vi "laneleftright411_temp.vi"() -> ()   [LabVIEW 2015]
uses:
  <vilib>/Analysis/6fits.llb/Curve Fitting Criteria.ctl
  <vilib>/Analysis/1siggen.llb/Ramp Pattern by Samples.vi
  <vilib>/Analysis/1siggen.llb/Ramp Pattern by Delta.vi
  G_ALL.vi
  <vilib>/Analysis/polynomials.llb/nth Derivative of Polynomial (DBL).vi
  <vilib>/Analysis/polynomials.llb/1D Polynomial Evaluation (DBL).vi
  G_LCM.vi
  <vilib>/Analysis/NI_AALBase.lvlib
  <vilib>/Analysis/NI_AALPro.lvlib
panel:
  out "y_ramp":dbl[](array[numeric])
  out "y_car":dbl[](array[numeric])
  out "x_car":dbl[](array[numeric])
  out "ynew":dbl[](array[numeric])
  out "x_rf":dbl[](array[numeric])
  out "y_rf":dbl[](array[numeric])
  out "y_rr":dbl[](array[numeric])
  out "x_rr":dbl[](array[numeric])
  out "x_lr":dbl[](array[numeric])
  out "y_lr":dbl[](array[numeric])
  out "x_left2":dbl[](array[numeric])
  out "leftfront":dbl[](array[numeric])
  out "af":dbl
  out "y_lf":dbl[](array[numeric])
  out "x_lf":dbl[](array[numeric])
  out "h_path":dbl[](array[numeric])
  out "x_path":dbl[](array[numeric])
  out "y_path":dbl[](array[numeric])
  out "gap":dbl
  out "Waveform Graph":dbl[](graph)
  out "x*y":dbl
  out "Array":dbl[](array[numeric])
  out "dy":dbl
  out "dx":dbl
  out "min value":dbl
  out "wgain":dbl[](array[numeric])
  out "min index":i32
  out "theta":dbl[](array[numeric])
  out "w":dbl[](array[numeric]) format="%.2f"
  out "y":dbl[](array[numeric])
  out "x":dbl[](array[numeric])
  out "r":dbl[](array[numeric])
  out "rout":dbl[](array[numeric])
  out "rin":dbl[](array[numeric])
  out "XY Graph":cluster{"Y":dbl[], "Y":dbl[]}[](graph)
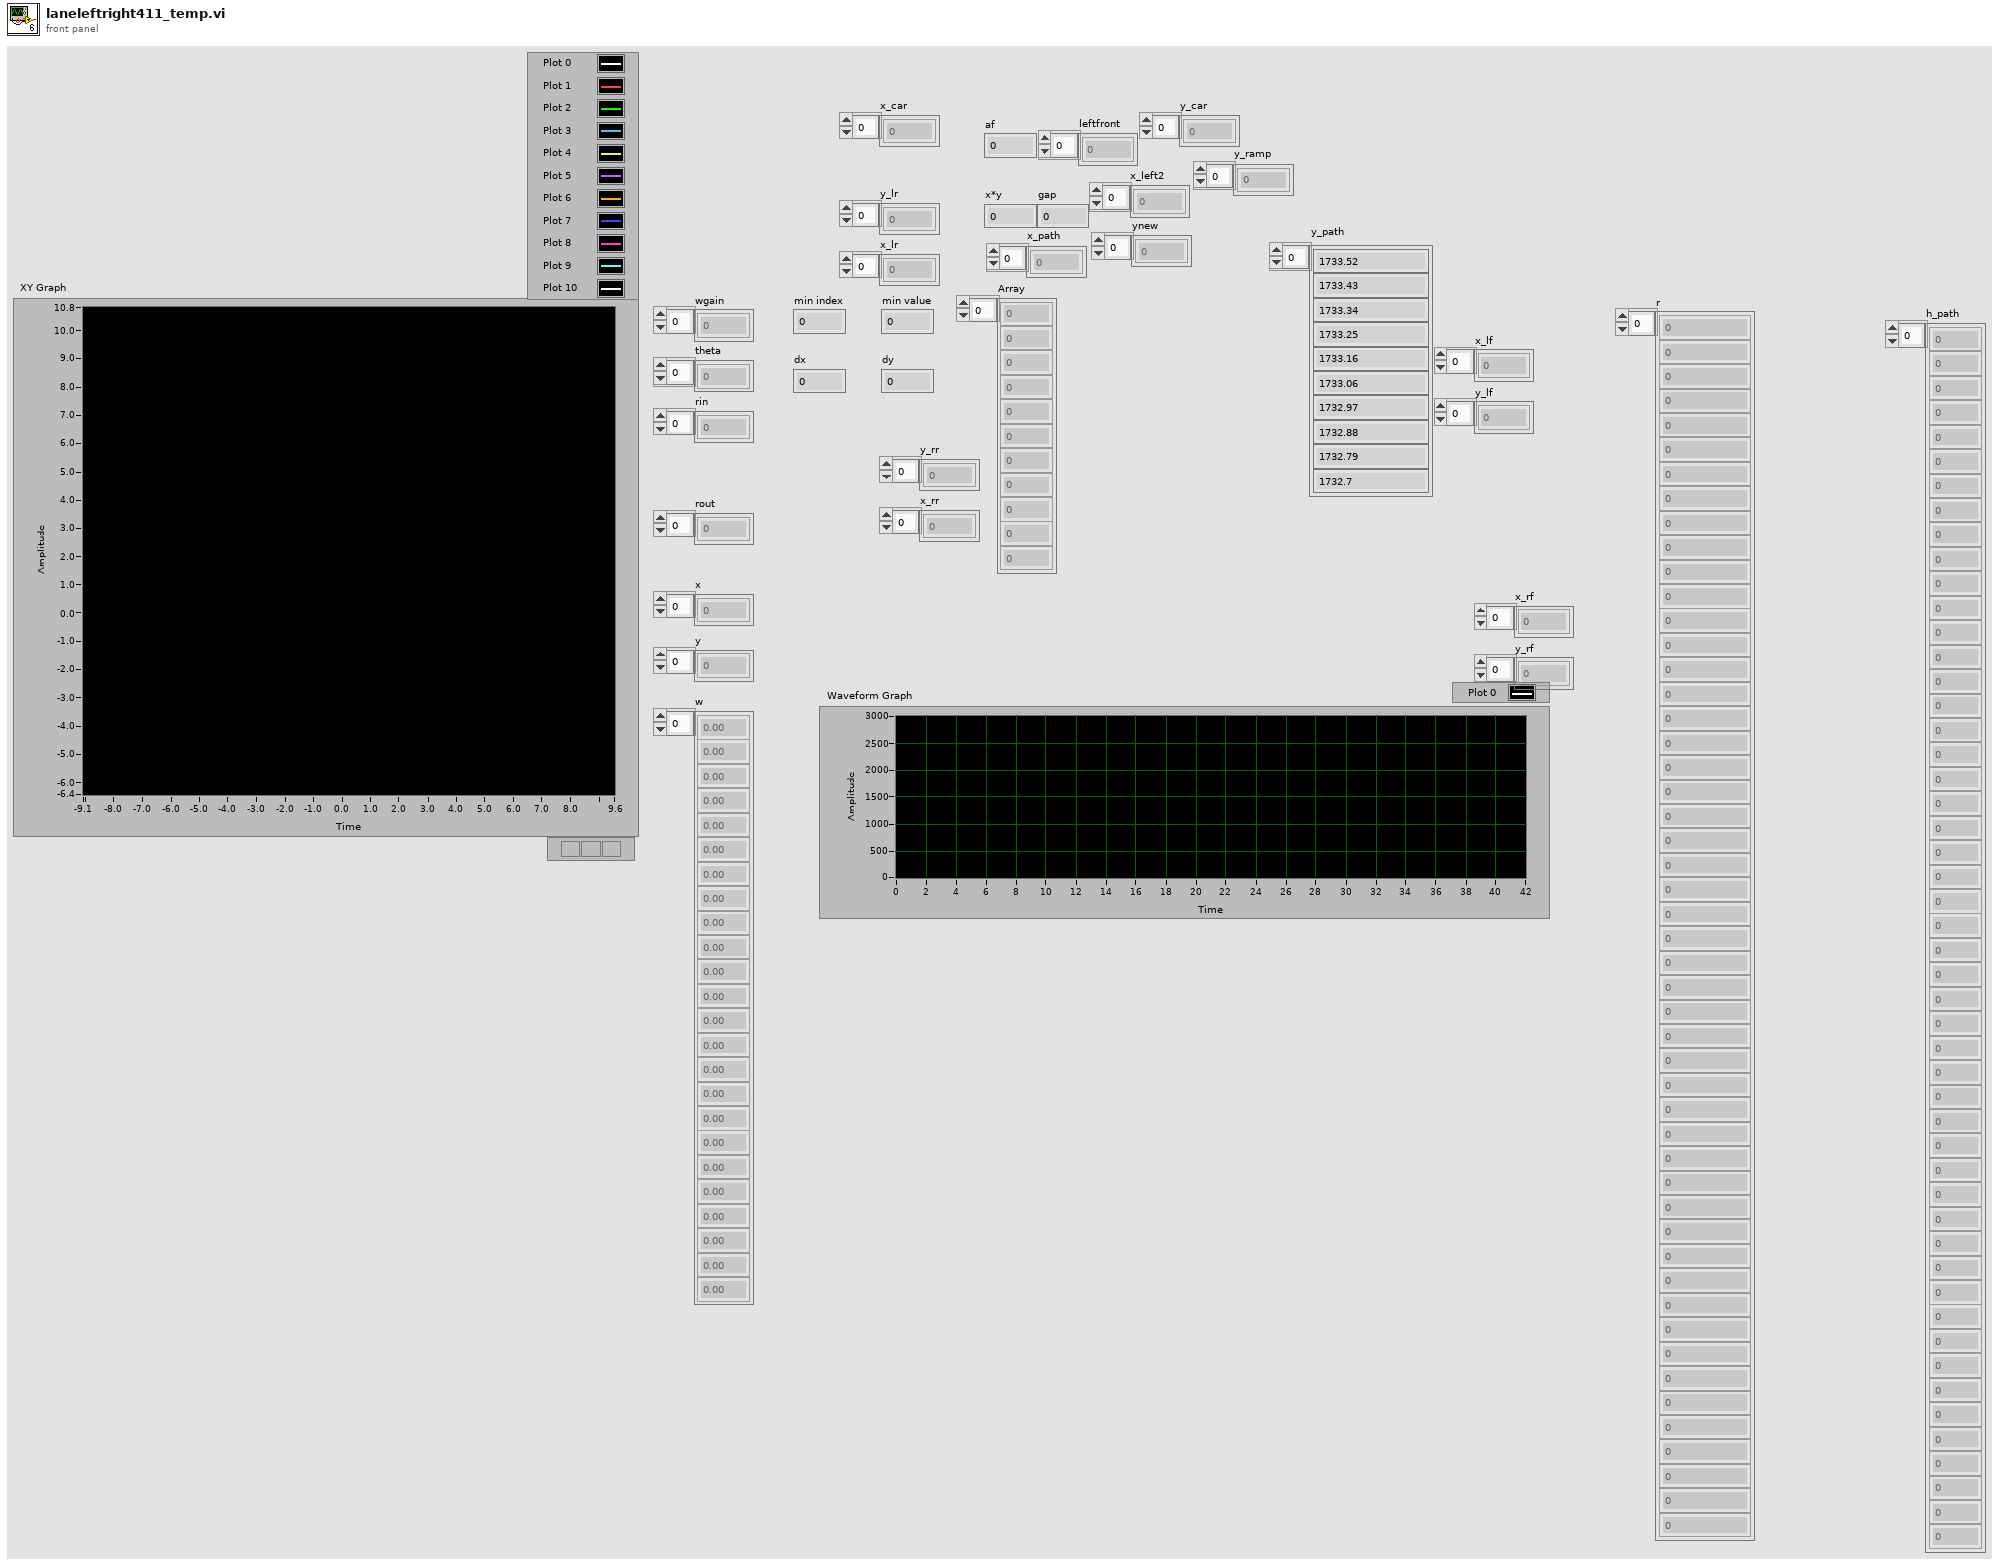
[diagram p1: front panel]
types:
  T1 = cluster{"C_Wheel base":dbl, "ratio_steer":dbl, "Overall width":dbl, "af":dbl, "turn radius":dbl, "eval":dbl, "ap":dbl, "an":dbl, "Vmax":dbl, "mu":dbl, "Vlast":dbl}
  T2 = typedef "NI_AALPro.lvlib/Curve Fitting Criteria.ctl" = u16
  T3 = cluster{"hash":i64, "sys time":i64, "size":i64, "x":dbl[], "y":dbl[], "point_flag":i32[]}
  T4 = cluster{"delta":bool, "Rotational position":dbl, "Rotational position":dbl}[]
  T5 = cluster{bool, "Rotational position":dbl, "Rotational position":dbl}[]
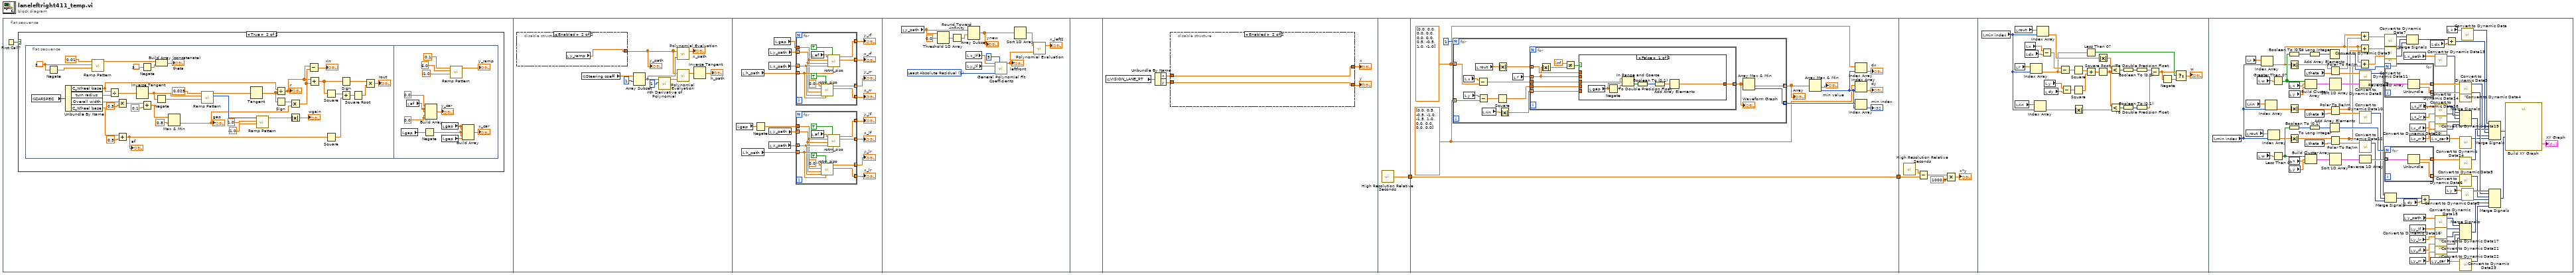
[diagram p0: block diagram]
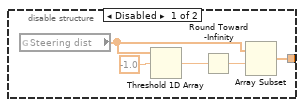
[diagram p3: hidden frame]
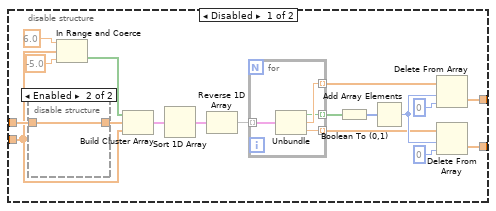
[diagram p4: hidden frame]
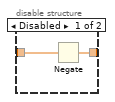
[diagram p5: hidden frame]
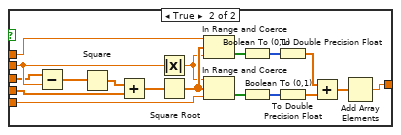
[diagram p6: hidden frame]
diagram:
  n1 = flat-sequence {
    tunnel: [w159] -> w2
    tunnel: w2 -> [w162]
    tunnel: [w162] -> w1
    tunnel: w1 -> [w223]
    frame #0 {
      n2 = First Call?() -> (First Call?: T/F=w3:bool)
      n3 = case shown="True" w3 {
        frame False {
        }
        frame True {
          n4 = flat-sequence {
            frame #0 {
              w27 = 3.141592653589793
              n5 = global read "G_ALL.vi" "CARSPEC"() -> (w45:T1)
              n6 = Negate(x=w27) -> (-x=w28:dbl)
              n7 = Unbundle By Name(w45) -> ("C_Wheel base"=w20:dbl, "turn radius"=w44:dbl, "Overall width"=w39:dbl, "C_Wheel base"=w6:dbl)
              n8 = call-poly <vilib>:"Ramp Pattern.vi"("start"=w28, "end"=w27, "delta"=0.01) -> ("Ramp Pattern"=w17:dbl[])  [unwired: 6 in, 2 out]
              n9 = Divide(x=w20, y=w44) -> (x/y=w43:dbl)
              n10 = Multiply(x=w39, y=0.5) -> (x*y=w19:dbl)
              n11 = Add(x=w6, y=0.5) -> (x+y=w4:dbl)
              "af" <- w4
              n12 = Inverse Tangent(1:w43) -> (0:w42:dbl)
              n13 = Negate(x=3.141592653589793) -> (-x=w14:dbl)
              n14 = Add(x=w19, y=0.1) -> (x+y=w9:dbl)
              n15 = Negate(x=w42) -> (-x=w10:dbl)
              n16 = Build Array (concatenate)(w17, w14) -> (→"theta":dbl[])
              n17 = Max & Min(x=w9, y=0.8) -> (min(x,y)=w8:dbl)  [unwired: 1 out]
              "gap" <- w8
              n18 = call-poly <vilib>:"Ramp Pattern.vi"("start"=w10, "end"=w42, "delta"=0.025) -> ("samples"=w25:i32, "Ramp Pattern"=w40:dbl[])  [unwired: 6 in, 1 out]
              n19 = Tangent(1:w40) -> (0:w37:dbl[])
              n20 = call-poly <vilib>:"Ramp Pattern.vi"("start"=-1.0, "end"=1.0, "samples"=w25) -> ("Ramp Pattern"=w22:dbl[])  [unwired: 7 in, 1 out]
              n21 = Divide(x=w20, y=w37) -> (x/y=w13:dbl[])
              "r" <- w13
              n22 = Sign(1:w37) -> (0:w36:dbl[])
              n23 = Multiply(x=w36, y=w8) -> (x*y=w35:dbl[])
              n24 = Absolute Value(x=w22) -> (abs(x)=→"wgain":dbl[])
              n25 = Subtract(x=w13, y=w35) -> (x-y=→"rin":dbl[])
              n26 = Add(x=w13, y=w35) -> (x+y=w31:dbl[])
              n27 = Square(x=w31) -> (x^2=w34:dbl[])
              n28 = Square(x=w4) -> (x^2=w33:dbl)
              n29 = Sign(1:w31) -> (0:w29:dbl[])
              n30 = Add(x=w34, y=w33) -> (x+y=w32:dbl[])
              n31 = Square Root(x=w32) -> (sqrt(x)=w30:dbl[])
              n32 = Multiply(x=w29, y=w30) -> (x*y=→"rout":dbl[])
            }
            frame #1 {
              w51 = 0.0 ("element")
              n33 = local read "gap"() -> (w58:dbl)
              n34 = local read "af"() -> (w53:dbl)
              n35 = Negate(x=w58) -> (-x=w56:dbl)
              n36 = Build Array(0.0 ("element"), w53, w53, w51, w51) -> (→"y_car":dbl[])
              n37 = local read "gap"() -> (w57:dbl)
              n38 = local read "gap"() -> (w55:dbl)
              n39 = call-poly <vilib>:"Ramp Pattern.vi"("start"=-1.0, "end"=6.0, "delta"=0.1) -> ("Ramp Pattern"=→"y_ramp":dbl[])  [unwired: 6 in, 2 out]
              n40 = Build Array(w57, w57, w56, w56, w55) -> (→"x_car":dbl[])
            }
          }
        }
      }
    }
    frame #1 {
      n41 = disable-structure shown="Enabled" {
        disable-tunnel: [w68 w73] -> w59
        frame Disabled {
          n42 = global read "G_ALL.vi" "Steering dist"() -> (w69:dbl[])
          n43 = Threshold 1D Array(2:-1.0 ("threshold y"), 3:w69) -> (0:w71:dbl)  [unwired: 1 in]
          n44 = Round Toward -Infinity(1:w71) -> (0:w70:dbl)
          n45 = Array Subset(array=w69, index=w70) -> (w68:dbl[])  [unwired: 1 in]
        }
        frame Enabled {
          n46 = local read "y_ramp"() -> (w73:dbl[])
        }
      }
      "y_path" <- w59
      n47 = global read "G_ALL.vi" "Steering coeff"() -> (w67:dbl[])
      n48 = Array Subset(array=w67, index=1) -> (w64:dbl[])  [unwired: 1 in]
      n49 = call-poly <vilib>:"nth Derivative of Polynomial.vi"("order"=1, "P(x)"=w64) -> ("Nth Derivative of P(x)"=w62:dbl[])  [unwired: 8 in, 1 out]
      n50 = call-poly <vilib>:"Polynomial Evaluation.vi"("P(x)"=w64, "A"=w59) -> ("P(A)"=→"x_path":dbl[])  [unwired: 1 out]
      n51 = call-poly <vilib>:"Polynomial Evaluation.vi"("P(x)"=w62, "A"=w59) -> ("P(A)"=w61:dbl[])  [unwired: 1 out]
      n52 = Inverse Tangent(1:w61) -> (0:→"h_path":dbl[])
    }
    frame #2 {
      n53 = local read "gap"() -> (w87:dbl)
      n54 = local read "h_path"() -> (w77:dbl[])
      n55 = local read "h_path"() -> (w88:dbl[])
      n56 = Negate(x=w87) -> (-x=w86:dbl)
      n57 = local read "y_path"() -> (w76:dbl[])
      n58 = local read "x_path"() -> (w75:dbl[])
      n59 = local read "y_path"() -> (w89:dbl[])
      n60 = local read "x_path"() -> (w90:dbl[])
      n61 = local read "gap"() -> (w74:dbl)
      n62 = for {
        tunnel: w75 -> [w97] mode=indexing
        tunnel: w76 -> [w96] mode=indexing
        tunnel: w77 -> [w98] mode=indexing
        tunnel: [w102] -> w78 mode=indexing
        tunnel: [w101] -> w79 mode=indexing
        tunnel: w74 -> [w95]
        tunnel: [w93] -> w80 mode=indexing
        tunnel: [w92] -> w81 mode=indexing
        n63 = local read "af"() -> (w99:dbl)
        n64 = call "rotm_siso.vi"("angle[rad]"=w98, "reverse"=TRUE, "y0"=w97, "x0"=w96, "y"=w95, "x"=0.0) -> ("y'"=w92:dbl, "x'"=w93:dbl)  [unwired: 4 in]
        n65 = call "rotm_siso.vi"("angle[rad]"=w98, "reverse"=TRUE, "y0"=w97, "x0"=w96, "y"=w95, "x"=w99) -> ("y'"=w101:dbl, "x'"=w102:dbl)  [unwired: 4 in]
      }
      "x_rf" <- w79
      "y_rf" <- w78
      "y_rr" <- w80
      "x_rr" <- w81
      n66 = for {
        tunnel: w90 -> [w109] mode=indexing
        tunnel: w89 -> [w108] mode=indexing
        tunnel: w88 -> [w110] mode=indexing
        tunnel: [w114] -> w85 mode=indexing
        tunnel: [w113] -> w84 mode=indexing
        tunnel: w86 -> [w107]
        tunnel: [w105] -> w83 mode=indexing
        tunnel: [w104] -> w82 mode=indexing
        n67 = local read "af"() -> (w111:dbl)
        n68 = call "rotm_siso.vi"("angle[rad]"=w110, "reverse"=TRUE, "y0"=w109, "x0"=w108, "y"=w107, "x"=0.0) -> ("y'"=w104:dbl, "x'"=w105:dbl)  [unwired: 4 in]
        n69 = call "rotm_siso.vi"("angle[rad]"=w110, "reverse"=TRUE, "y0"=w109, "x0"=w108, "y"=w107, "x"=w111) -> ("y'"=w113:dbl, "x'"=w114:dbl)  [unwired: 4 in]
      }
      "x_lf" <- w84
      "y_lf" <- w85
      "y_lr" <- w83
      "x_lr" <- w82
    }
    frame #3 {
      w122 = T2 1 items=["Least Square", "Least Absolute Residual", "Bisquare"] ("method")
      n70 = local read "y_path"() -> (w117:dbl[])
      n71 = Threshold 1D Array(2:0.0 ("threshold y"), 3:w117) -> (0:w118:dbl)  [unwired: 1 in]
      n72 = Round Toward -Infinity(1:w118) -> (0:w116:dbl)
      n73 = local read "x_lf"() -> (w125:dbl[])
      n74 = local read "y_lf"() -> (w120:dbl[])
      n75 = Array Subset(array=w117, index=w116) -> (w115:dbl[])  [unwired: 1 in]
      "ynew" <- w115
      n76 = call <vilib>:"General Polynomial Fit Coefficients.vi"("Y"=w125, "polynomial order"=5, "X"=w120, "method"=w122) -> ("Polynomial Coefficients"=w124:dbl[])  [unwired: 10 in, 1 out]
      "leftfront" <- w124
      n77 = Sort 1D Array(array=w115) -> (sorted array=w121:dbl[])
      n78 = call-poly <vilib>:"Polynomial Evaluation.vi"("P(x)"=w124, "A"=w121) -> ("P(A)"=→"x_left2":dbl[])  [unwired: 1 out]
    }
    frame #4 {
    }
    frame #5 {
      n79 = global read "G_LCM.vi" "VISION_LANE_PT"() -> (w131:T3)
      n80 = Unbundle By Name(w131) -> ("x"=w130:dbl[], "y"=w129:dbl[])
      n81 = disable-structure shown="Enabled" {
        disable-tunnel: w130 -> [w148 w158]
        disable-tunnel: [w146 w157] -> w127
        disable-tunnel: [w145 w158] -> w128
        disable-tunnel: w129 -> [w142 w157]
        frame Disabled {
          n82 = disable-structure shown="Enabled" {
            disable-tunnel: w148 -> [w151 w152]
            disable-tunnel: [w150 w152] -> w149
            frame Disabled {
              n83 = Negate(x=w151) -> (-x=w150:dbl[])
            }
            frame Enabled {
            }
          }
          n84 = In Range and Coerce(upper limit=6.0 ("delta"), x=w142, lower limit=-5.0) -> (In Range?=w140:bool[])  [unwired: 1 out]
          n85 = Build Cluster Array(w140, w149, w142) -> (w138:T4)
          n86 = Sort 1D Array(array=w138) -> (sorted array=w139:T4)
          n87 = Reverse 1D Array(array=w139) -> (reversed array=w135:T4)
          n88 = for {
            tunnel: w135 -> [w156] mode=indexing
            tunnel: [w155] -> w133 mode=indexing
            tunnel: [w154] -> w132 mode=indexing
            tunnel: [w153] -> w143 mode=indexing
            n89 = Unbundle(w156) -> ("delta"=w153:bool, "Rotational position"=w155:dbl, "Rotational position"=w154:dbl)
          }
          n90 = Boolean To (0,1)(Boolean=w143) -> (0, 1=w136:i16[])
          n91 = Add Array Elements(numeric array=w136) -> (sum=w144:i16)
          n92 = Delete From Array(array=w133, length=w144, index=0) -> (deleted portion=w145:dbl[])  [unwired: 1 out]
          n93 = Delete From Array(array=w132, length=w144, index=0) -> (deleted portion=w146:dbl[])  [unwired: 1 out]
        }
        frame Enabled {
        }
      }
      "x" <- w128
      "y" <- w127
    }
    frame #6 {
      n94 = call <vilib>:"High Resolution Relative Seconds.vi"() -> ("relative seconds"=w159:dbl)
    }
    frame #7 {
      w160 = dbl[] [0.0, 0.5, -0.5, -1.0, -1.5, 1.0, 0.0, 0.0, 0.0, 0.0]
      w161 = dbl[] [0.0, 0.0, 0.0, 0.0, 0.0, 0.0, 0.5, -0.5, 1.0, -1.0]
      n95 = for {
        N: 1 -> [_]
        tunnel: [w172] -> w170 mode=indexing
        tunnel: w161 -> [w177] mode=indexing
        tunnel: w160 -> [w175] mode=indexing
        tunnel: [w174] -> w169 mode=indexing
        n96 = local read "x"() -> (w179:dbl[])
        n97 = local read "y"() -> (w176:dbl[])
        n98 = local read "rout"() -> (w183:dbl[])
        n99 = Subtract(x=w179, y=w177) -> (x-y=w178:dbl[])
        n100 = Subtract(x=w176, y=w175) -> (x-y=w173:dbl[])
        n101 = local read "rin"() -> (w181:dbl[])
        n102 = Square(x=w173) -> (x^2=w184:dbl[])
        n103 = Absolute Value(x=w183) -> (abs(x)=w182:dbl[])
        n104 = Absolute Value(x=w181) -> (abs(x)=w180:dbl[])
        n105 = local read "r"() -> (w185:dbl[])
        n106 = for {
          tunnel: w185 -> [w189] mode=indexing
          tunnel: w184 -> [w194]
          tunnel: w182 -> [w193] mode=indexing
          tunnel: w180 -> [w192] mode=indexing
          tunnel: [w191] -> w171 mode=indexing
          tunnel: w178 -> [w190]
          n107 = Absolute Value(x=w189) -> (abs(x)=w186:dbl)
          n108 = Not Equal?(x=inf, y=w186) -> (x != y?=w187:bool)
          n109 = case shown="False" w187 {
            tunnel: w194 -> [_ w217]
            tunnel: w193 -> [_ w214]
            tunnel: w192 -> [_ w213]
            tunnel: w189 -> [_ w209]
            tunnel: [w195 w206] -> w191
            tunnel: w190 -> [w201 w205]
            frame False {
              n110 = local read "gap"() -> (w200:dbl)
              n111 = Negate(x=w200) -> (-x=w199:dbl)
              n112 = In Range and Coerce(upper limit=w200, x=w201, lower limit=w199) -> (In Range?=w197:bool[])  [unwired: 1 out]
              n113 = Boolean To (0,1)(Boolean=w197) -> (0, 1=w198:i16[])
              n114 = To Double Precision Float(number=w198) -> (double precision float=w196:dbl[])
              n115 = Add Array Elements(numeric array=w196) -> (sum=w195:dbl)
            }
            frame True {
              n116 = Subtract(x=w205, y=w209) -> (x-y=w219:dbl[])
              n117 = Square(x=w219) -> (x^2=w218:dbl[])
              n118 = Add(x=w218, y=w217) -> (x+y=w216:dbl[])
              n119 = Absolute Value(x=w209) -> (abs(x)=w210:dbl)
              n120 = Square Root(x=w216) -> (sqrt(x)=w215:dbl[])
              n121 = In Range and Coerce(upper limit=w214, x=w215, lower limit=w210) -> (In Range?=w204:bool[])  [unwired: 1 out]
              n122 = In Range and Coerce(upper limit=w210, x=w215, lower limit=w213) -> (In Range?=w203:bool[])  [unwired: 1 out]
              n123 = Boolean To (0,1)(Boolean=w204) -> (0, 1=w212:i16[])
              n124 = Boolean To (0,1)(Boolean=w203) -> (0, 1=w211:i16[])
              n125 = To Double Precision Float(number=w212) -> (double precision float=w208:dbl[])
              n126 = To Double Precision Float(number=w211) -> (double precision float=w207:dbl[])
              n127 = Add(x=w208, y=w207) -> (x+y=w202:dbl[])
              n128 = Add Array Elements(numeric array=w202) -> (sum=w206:dbl)
            }
          }
        }
        "Waveform Graph" <- w171
        n129 = Array Max & Min(array=w171) -> (min value=w172:dbl, min index (indices)=w174:i32)  [unwired: 2 out]
      }
      "Array" <- w170
      n130 = Array Max & Min(array=w170) -> (min value=→"min value":dbl, min index (indices)=w164:i32)  [unwired: 2 out]
      n131 = Index Array(array=w161, index=w164) -> (element=→"dx":dbl)
      n132 = Index Array(array=w160, index=w164) -> (element=→"dy":dbl)
      n133 = Index Array(array=w169, index=w164) -> (element=→"min index":i32)
    }
    frame #8 {
      n134 = call <vilib>:"High Resolution Relative Seconds.vi"() -> ("relative seconds"=w224:dbl)
      n135 = Subtract(x=w224, y=w223) -> (x-y=w222:dbl)
      n136 = Multiply(x=w222, y=1000.0) -> (x*y=→"x*y":dbl)
    }
    frame #9 {
      n137 = local read "min index"() -> (w237:i32)
      n138 = local read "rout"() -> (w241:dbl[])
      n139 = local read "r"() -> (w229:dbl[])
      n140 = local read "rin"() -> (w247:dbl[])
      n141 = local read "x"() -> (w236:dbl[])
      n142 = local read "dx"() -> (w234:dbl)
      n143 = Index Array(array=w229, index=w237) -> (element=w228:dbl)
      n144 = Index Array(array=w247, index=w237) -> (element=w253:dbl)
      n145 = Index Array(array=w241, index=w237) -> (element=w242:dbl)
      n146 = Subtract(x=w236, y=w234) -> (x-y=w235:dbl[])
      n147 = local read "y"() -> (w232:dbl[])
      n148 = local read "dy"() -> (w233:dbl)
      n149 = Subtract(x=w235, y=w228) -> (x-y=w243:dbl[])
      n150 = Subtract(x=w232, y=w233) -> (x-y=w231:dbl[])
      n151 = Square(x=w243) -> (x^2=w244:dbl[])
      n152 = Square(x=w231) -> (x^2=w245:dbl[])
      n153 = Absolute Value(x=w253) -> (abs(x)=w254:dbl)
      n154 = Less Than 0?(x=w228) -> (x < 0?=w230:bool)
      n155 = Add(x=w244, y=w245) -> (x+y=w246:dbl[])
      n156 = Absolute Value(x=w242) -> (abs(x)=w240:dbl)
      n157 = Square Root(x=w246) -> (sqrt(x)=w239:dbl[])
      n158 = Less?(x=w240, y=w239) -> (x < y?=w238:bool[])
      n159 = Less?(x=w239, y=w254) -> (x < y?=w248:bool[])
      n160 = Boolean To (0,1)(Boolean=w238) -> (0, 1=w251:i16[])
      n161 = Boolean To (0,1)(Boolean=w248) -> (0, 1=w249:i16[])
      n162 = To Double Precision Float(number=w251) -> (double precision float=w252:dbl[])
      n163 = To Double Precision Float(number=w249) -> (double precision float=w250:dbl[])
      n164 = Subtract(x=w252, y=w250) -> (x-y=w225:dbl[])
      n165 = Negate(x=w225) -> (-x=w226:dbl[])
      n166 = Select(t=w225, s=w230, f=w226) -> (s? t:f=→"w":dbl[])
    }
    frame #10 {
      n167 = local read "min index"() -> (w299:i32)
      n168 = local read "r"() -> (w306:dbl[])
      n169 = local read "rin"() -> (w305:dbl[])
      n170 = local read "rout"() -> (w300:dbl[])
      n171 = local read "w"() -> (w329:dbl[])
      n172 = local read "w"() -> (w328:dbl[])
      n173 = Index Array(array=w306, index=w299) -> (element=w295:dbl)
      n174 = Index Array(array=w305, index=w299) -> (element=w304:dbl)
      n175 = Index Array(array=w300, index=w299) -> (element=w301:dbl)
      n176 = Greater Than 0?(x=w329) -> (x > 0?=w343:bool[])
      n177 = Less Than 0?(x=w328) -> (x < 0?=w320:bool[])
      n178 = Boolean To (0,1)(Boolean=w343) -> (0, 1=w342:i16[])
      n179 = Absolute Value(x=w295) -> (abs(x)=w313:dbl)
      n180 = Absolute Value(x=w304) -> (abs(x)=w308:dbl)
      n181 = Boolean To (0,1)(Boolean=w320) -> (0, 1=w321:i16[])
      n182 = Absolute Value(x=w301) -> (abs(x)=w297:dbl)
      n183 = local read "x"() -> (w344:dbl[])
      n184 = local read "y"() -> (w330:dbl[])
      n185 = local read "x"() -> (w319:dbl[])
      n186 = local read "y"() -> (w327:dbl[])
      n187 = local read "theta"() -> (w314:dbl[])
      n188 = Build Cluster Array(w343, w344, w330) -> (w340:T5)
      n189 = local read "theta"() -> (w307:dbl[])
      n190 = local read "theta"() -> (w298:dbl[])
      n191 = Build Cluster Array(w320, w319, w327) -> (w323:T5)
      n192 = To Long Integer(number=w342) -> (32bit integer=w341:i32[])
      n193 = To Long Integer(number=w321) -> (32bit integer=w322:i32[])
      n194 = Add Array Elements(numeric array=w341) -> (sum=w338:i32)
      n195 = Add Array Elements(numeric array=w322) -> (sum=w325:i32)
      n196 = Polar To Re/Im(2:w314, 3:w313) -> (0:w310:dbl[], 1:w312:dbl[])
      n197 = Sort 1D Array(array=w340) -> (sorted array=w339:T5)
      n198 = Polar To Re/Im(2:w307, 3:w308) -> (0:w302:dbl[], 1:w309:dbl[])
      n199 = Polar To Re/Im(2:w298, 3:w297) -> (0:w293:dbl[], 1:w296:dbl[])
      n200 = Sort 1D Array(array=w323) -> (sorted array=w324:T5)
      n201 = Add(x=w295, y=w312) -> (x+y=w311:dbl[])
      n202 = Add(x=w295, y=w309) -> (x+y=w303:dbl[])
      n203 = Add(x=w295, y=w296) -> (x+y=w294:dbl[])
      n204 = call "Convert to Dynamic Data8"("Array"=w310) -> ("Dynamic Data Type"=w286:dynamicdata)  [unwired: 3 in]
      n205 = Reverse 1D Array(array=w339) -> (reversed array=w337:T5)
      n206 = call "Convert to Dynamic Data10"("Array"=w302) -> ("Dynamic Data Type"=w285:dynamicdata)  [unwired: 3 in]
      n207 = call "Convert to Dynamic Data12"("Array"=w293) -> ("Dynamic Data Type"=w284:dynamicdata)  [unwired: 3 in]
      n208 = Reverse 1D Array(array=w324) -> (reversed array=w326:T5)
      n209 = call "Convert to Dynamic Data7"("Array"=w311) -> ("Dynamic Data Type"=w292:dynamicdata)  [unwired: 3 in]
      n210 = call "Convert to Dynamic Data9"("Array"=w303) -> ("Dynamic Data Type"=w291:dynamicdata)  [unwired: 3 in]
      n211 = call "Convert to Dynamic Data11"("Array"=w294) -> ("Dynamic Data Type"=w290:dynamicdata)  [unwired: 3 in]
      n212 = for {
        N: w338 -> [_]
        tunnel: w337 -> [w355] mode=indexing
        tunnel: [w354] -> w335 mode=indexing
        tunnel: [w353] -> w332 mode=indexing
        n213 = Unbundle(w355) -> ("Rotational position"=w354:dbl, "Rotational position"=w353:dbl)  [unwired: 1 out]
      }
      n214 = for {
        N: w325 -> [_]
        tunnel: w326 -> [w352] mode=indexing
        tunnel: [w351] -> w318 mode=indexing
        tunnel: [w350] -> w316 mode=indexing
        n215 = Unbundle(w352) -> ("Rotational position"=w351:dbl, "Rotational position"=w350:dbl)  [unwired: 1 out]
      }
      n216 = Merge Signals(w286, w285, w284) -> (w283:dynamicdata)
      n217 = local read "x_path"() -> (w280:dbl[])
      n218 = local read "dy"() -> (w282:dbl)
      n219 = local read "y_path"() -> (w268:dbl[])
      n220 = Merge Signals(w292, w291, w290) -> (w289:dynamicdata)
      n221 = local read "x_rf"() -> (w265:dbl[])
      n222 = local read "x_rr"() -> (w266:dbl[])
      n223 = local read "y_lf"() -> (w274:dbl[])
      n224 = local read "y_lr"() -> (w267:dbl[])
      n225 = local read "y_rf"() -> (w261:dbl[])
      n226 = local read "y_rr"() -> (w262:dbl[])
      n227 = local read "x_lf"() -> (w278:dbl[])
      n228 = local read "x_lr"() -> (w270:dbl[])
      n229 = Add(x=w283, y=w282) -> (x+y=w281:dynamicdata)
      n230 = local read "dx"() -> (w288:dbl)
      n231 = local read "x_car"() -> (w256:dbl[])
      n232 = local read "y_car"() -> (w258:dbl[])
      n233 = call "Convert to Dynamic Data13"("Array"=w280) -> ("Dynamic Data Type"=w279:dynamicdata)  [unwired: 3 in]
      n234 = call "Convert to Dynamic Data14"("Array"=w278) -> ("Dynamic Data Type"=w277:dynamicdata)  [unwired: 3 in]
      n235 = call "Convert to Dynamic Data18"("Array"=w270) -> ("Dynamic Data Type"=w269:dynamicdata)  [unwired: 3 in]
      n236 = call "Convert to Dynamic Data19"("Array"=w265) -> ("Dynamic Data Type"=w264:dynamicdata)  [unwired: 3 in]
      n237 = call "Convert to Dynamic Data20"("Array"=w266) -> ("Dynamic Data Type"=w263:dynamicdata)  [unwired: 3 in]
      n238 = call "Convert to Dynamic Data15"("Array"=w268) -> ("Dynamic Data Type"=w273:dynamicdata)  [unwired: 3 in]
      n239 = call "Convert to Dynamic Data16"("Array"=w274) -> ("Dynamic Data Type"=w275:dynamicdata)  [unwired: 3 in]
      n240 = call "Convert to Dynamic Data17"("Array"=w267) -> ("Dynamic Data Type"=w271:dynamicdata)  [unwired: 3 in]
      n241 = call "Convert to Dynamic Data21"("Array"=w261) -> ("Dynamic Data Type"=w260:dynamicdata)  [unwired: 3 in]
      n242 = call "Convert to Dynamic Data22"("Array"=w262) -> ("Dynamic Data Type"=w259:dynamicdata)  [unwired: 3 in]
      n243 = Add(x=w289, y=w288) -> (x+y=w287:dynamicdata)
      n244 = local read "y"() -> (w345:dbl[])
      n245 = local read "x"() -> (w346:dbl[])
      n246 = Merge Signals(w279, w277, w269, w264, w263) -> (w276:dynamicdata)
      n247 = Merge Signals(w273, w275, w271, w260, w259) -> (w272:dynamicdata)
      n248 = call "Convert to Dynamic Data3"("Array"=w335) -> ("Dynamic Data Type"=w334:dynamicdata)  [unwired: 3 in]
      n249 = call "Convert to Dynamic Data4"("Array"=w332) -> ("Dynamic Data Type"=w331:dynamicdata)  [unwired: 3 in]
      n250 = call "Convert to Dynamic Data24"("Array"=w256) -> ("Dynamic Data Type"=w255:dynamicdata)  [unwired: 3 in]
      n251 = call "Convert to Dynamic Data5"("Array"=w318) -> ("Dynamic Data Type"=w317:dynamicdata)  [unwired: 3 in]
      n252 = call "Convert to Dynamic Data6"("Array"=w316) -> ("Dynamic Data Type"=w315:dynamicdata)  [unwired: 3 in]
      n253 = call "Convert to Dynamic Data23"("Array"=w258) -> ("Dynamic Data Type"=w257:dynamicdata)  [unwired: 3 in]
      n254 = call "Convert to Dynamic Data2"("Array"=w345) -> ("Dynamic Data Type"=w349:dynamicdata)  [unwired: 3 in]
      n255 = call "Convert to Dynamic Data"("Array"=w346) -> ("Dynamic Data Type"=w348:dynamicdata)  [unwired: 3 in]
      n256 = Merge Signals(w348, w334, w317, w287, w276, w255) -> (w336:dynamicdata)
      n257 = Merge Signals(w349, w331, w315, w281, w272, w257) -> (w333:dynamicdata)
      n258 = call "Build XY Graph"("Y Input"=w333, "X Input"=w336) -> ("XY Graph"=→"XY Graph":cluster{"X":dbl[], "Y":dbl[]}[])  [unwired: 8 in, 1 out]
    }
  }
